vi "GetCurrent.vi"(8 "Error In":errorcluster, 11 "object in":refnum<class "IEnumerator.lvclass">) -> (0 "Error Out":errorcluster, 2 "Return(LabVIEW Object)":refnum<class>, 3 "object out":refnum<class "IEnumerator.lvclass">)   [LabVIEW 2020, in "IEnumerator.lvclass"]
uses:
  IEnumerator.lvclass
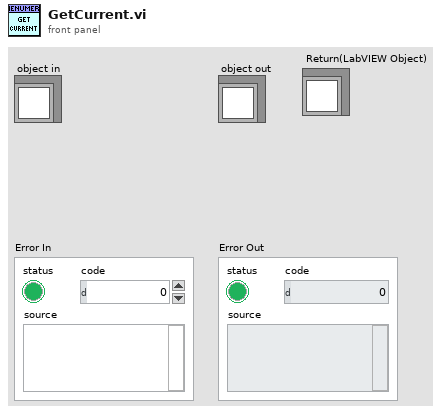
[diagram p1: front panel]
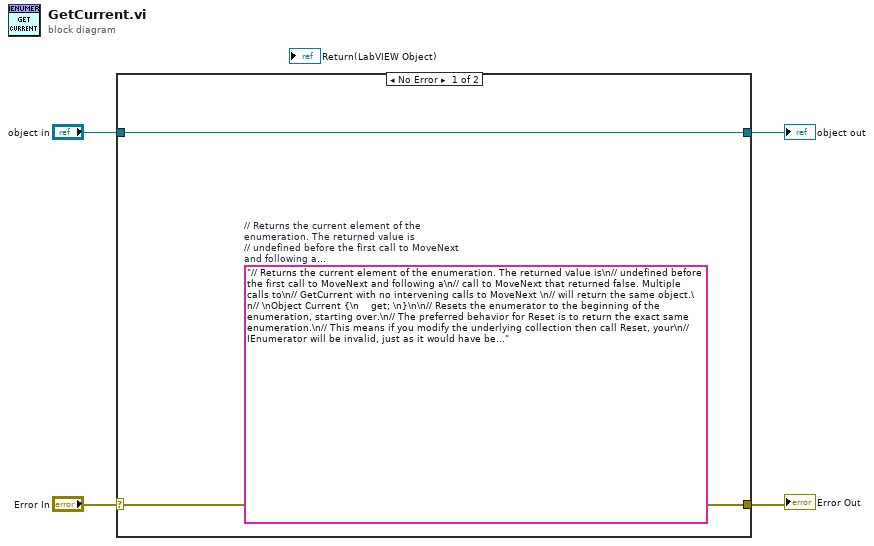
[diagram p0: block diagram]
diagram:
  (unwired) "// Returns the current element of the enumeration. The returned value is\n// undefined before the first call to MoveNext and following a\n// call to MoveNext that returned false. Multiple calls to\n// GetCurrent with no intervening calls to MoveNext \n// will return the same object.\n// \nObject Current {\n    get; \n}\n\n// Resets the enumerator to the beginning of the enumeration, starting over.\n// The preferred behavior for Reset is to return the exact same enumeration.\n// This means if you modify the underlying collection then call Reset, your\n// IEnumerator will be invalid, just as it would have been if you had called\n// MoveNext or Current.\n//\nvoid Reset()"  # // Returns the current element of the enumeration. The returned value is // undefined before the first call to MoveNext and following a // call to MoveNext that returned false. Multiple calls to // GetCurrent with no intervening calls to MoveNext  // will return the same object. //  Object Current {     get;  }  // Resets the enumerator to the beginning of the enumeration, starting over. // The preferred behavior for Reset is to return the exact same enumeration. // This means if you modify the underlying collection then call Reset, your // IEnumerator will be invalid, just as it would have been if you had called // MoveNext or Current. // void Reset()
  n1 = case shown="No Error" "Error In" {
    selector: "Error In" -> [w6 w8]
    tunnel: [w6 w8] -> w3
    tunnel: [w5 w7] -> w1
    tunnel: "object in" -> [w5 w7]
    frame No Error {
    }
    frame Error {
    }
  }
  "Error Out" <- w3
  "object out" <- w1
